vi "Read.vi"(8 "error in (no error)":errorcluster, 11 "PVConnection in":refnum<class "SVConnection.lvclass">) -> (0 "error out":errorcluster, 2 "PV":refnum<class "PV.lvclass">, 3 "PVConnection out":refnum<class "SVConnection.lvclass">)   [LabVIEW 2013, in "CS++ProcessVariables.lvlib" / "SVConnection.lvclass"]
doc: "Read a process varibale."
uses:
  SVConnection.lvclass
  ProcessVariable/PV.lvclass
  SVConnection.lvclass/SVConnection.ctl
  PVConnection/PVConnection.lvclass/PVConnection.ctl
  ProcessVariable/PV.lvclass/PV.ctl
  ProcessVariable/Write PV URL.vi
  ProcessVariable/Write Data.vi
  ProcessVariable/Write Error.vi
  ProcessVariable/Write Timestamp.vi
  ProcessVariable/Write status.vi
  ProcessVariable/Write Quality.vi
  PVConnection/PVConnection.lvclass
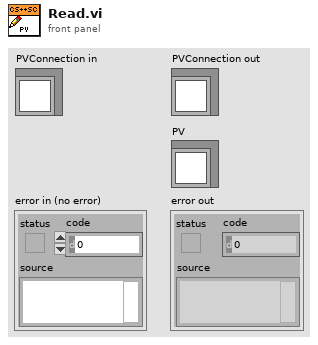
[diagram p1: front panel]
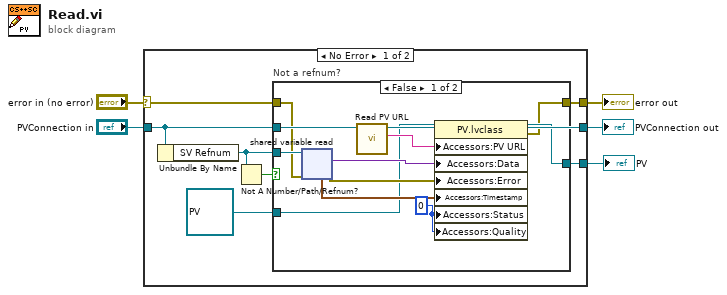
[diagram p0: block diagram]
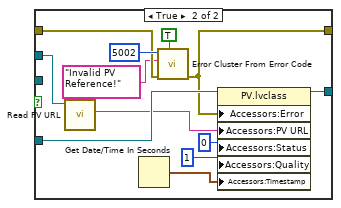
[diagram p2: hidden frame]
diagram:
  n1 = case shown="No Error" "error in (no error)" {
    selector: "error in (no error)" -> [w9 w36]
    tunnel: [w12 w36] -> w2
    tunnel: [w8 w37] -> w3
    tunnel: "PVConnection in" -> [w8 w37]
    tunnel: [w7 _] -> w1
    frame No Error {
      n2 = Unbundle By Name(w8) -> ("SV Refnum"=w10:refnum<k21>)
      n3 = Not A Number/Path/Refnum?(number/path/refnum=w10) -> (NaN/Path/Refnum?=w11:bool)
      n4 = case "Not a refnum?" shown="False" w11 {
        tunnel: w10 -> [w23 _]
        tunnel: w9 -> [w22 w33]
        tunnel: [w14 w28] -> w12
        tunnel: w8 -> [w21 w30]
        tunnel: [w16 w29] -> w7
        tunnel: refnum<class "PV.lvclass"> refnum ("CS++ProcessVariables.lvlib:PV.lvclass") -> [w13 w31]
        frame False {
          w17 = u32 0 ("status")
          n5 = shared-variable-read(w23, w22) -> (w15:errorcluster, w19:variant, w18:timestamp)  [unwired: 1 out]
          n6 = call "Read PV URL.vi"("PVConnection in"=w21) -> ("PV URL"=w20:string)  [unwired: 8 in, 2 out]
          n7 = property class="PV.lvclass"(reference=w13, "Accessors:PV URL"=w20, "Accessors:Data"=w19, "Accessors:Error"=w15, "Accessors:Timestamp"=w18, "Accessors:Status"=w17, "Accessors:Quality"=w17) -> (reference out=w16:refnum<class "PV.lvclass">, error out=w14:errorcluster)  [unwired: 1 in]
        }
        frame True {
          n8 = call "Read PV URL.vi"("PVConnection in"=w30) -> ("PV URL"=w27:string)  [unwired: 8 in, 2 out]
          n9 = Get Date/Time In Seconds() -> (seconds since 1Jan1904=w24:timestamp)
          n10 = call <vilib>:"Error Cluster From Error Code.vi"("show call chain? (False)"=TRUE, "error in (no error)"=w33, "error message (\"\")"="Invalid PV Reference!" ("error message (\"\")"), "error code (0)"=5002) -> ("error out"=w28:errorcluster)  [unwired: 5 in]
          n11 = property class="PV.lvclass"(reference=w31, "Accessors:Error"=w28, "Accessors:PV URL"=w27, "Accessors:Status"=u32 0 ("status"), "Accessors:Quality"=u64 1 ("quality"), "Accessors:Timestamp"=w24) -> (reference out=w29:refnum<class "PV.lvclass">)  [unwired: 1 in, 1 out]
        }
      }
    }
    frame Error {
    }
  }
  "error out" <- w2
  "PVConnection out" <- w3
  "PV" <- w1
